vi "3A control PWM.vi"() -> ()   [LabVIEW 2011]
uses:
  <vilib>/FPGAPlugInAG/cRIO-9113/niLvFpga_Open_cRIO-9113.vi
  <vilib>/Utility/error.llb/Error Cluster From Error Code.vi
  <vilib>/rvi/errors/niLvFpgaAdjustHostInterfaceError.vi
  <vilib>/FPGAPlugInAG/cRIO-9113/niLvFpga_Close_cRIO-9113.vi
  <vilib>/rvi/interface/nirviOpenFPGA/nirviOpenFPGA.xnode
  FPGA Bitfiles/SailBot_FPGATarget_PWM_D13D3FCE.lvbitx
  <vilib>/rvi/interface/nirviReadWriteControl/nirviReadWriteControl.xnode
  <vilib>/rvi/interface/nirviCloseFPGA/nirviCloseFPGA.xnode
  NiFpgaLv.dll
panel:
  in  "CCW Servo Angle (radians)":dbl(slide) scale=1.57..-1.57
  in  "stop":bool
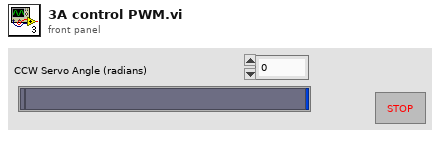
[diagram p1: front panel]
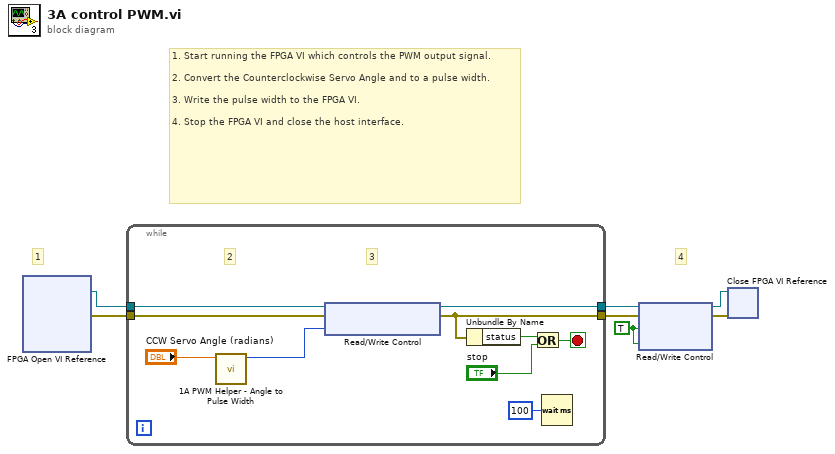
[diagram p0: block diagram]
diagram:
  w1 = TRUE ("stop")
  # "1. Start running the FPGA VI which controls the PWM output signal.\n\n2. Convert the Counterclockwise Servo Angle and to a pulse width.\n\n3. Write the pulse width to the FPGA VI.\n\n4. Stop the FPGA VI and close the host interface."
  # "4"
  # "1"
  n1 = xnode "FPGA Open VI Reference"() -> ("FPGA VI Reference Out"=w7:refnum<k20>, "error out"=w6:errorcluster)  [unwired: 2 in]
  n2 = while {
    tunnel: w7 -> [w16]
    tunnel: w6 -> [w13]
    tunnel: [w11] -> w2
    tunnel: [w12] -> w4
    stop <- w9 stop-if-true
    # "3"
    # "2"
    n3 = call "1A PWM Helper - Angle to Pulse Width.vi"("ccw servo angle (radians)"="CCW Servo Angle (radians)") -> ("pulse width (us)"=w14:u32)  [unwired: 10 in]
    n4 = xnode "Read/Write Control"("FPGA VI Reference In"=w16, "error in"=w13, "pulse width (uSec)"=w14) -> ("FPGA VI Reference Out"=w12:refnum<k20>, "error out"=w11:errorcluster)
    n5 = Unbundle By Name(w11) -> ("status"=w10:bool)
    n6 = Or(x=w10, y="stop") -> (x .or. y?=w9:bool)
    n7 = Wait (ms)(milliseconds to wait=u32 100 ("Count(mSec)")) -> ()  [unwired: 1 out]
  }
  n8 = xnode "Read/Write Control"("FPGA VI Reference In"=w4, "error in"=w2, "stop PWM"=w1, "stop blink"=w1) -> ("FPGA VI Reference Out"=w5:refnum<k20>, "error out"=w3:errorcluster)
  n9 = xnode "Close FPGA VI Reference"("FPGA VI Reference In"=w5, "error in"=w3) -> ()  [unwired: 1 out]
